vi "AccelerometerSample6.vi"(0 "Output type":i16=1, 1 "Period (ms)":i32=5) -> (2 "Ticks":u64, 3 "FIFO full":bool, 4 "Timeouted":bool)   [LabVIEW 2018]
uses:
  <vilib>/rvi/Emulation/niFpgaGetClockAttributes.vi
  <vilib>/rvi/Emulation/niFpgaSctlEmulationGetInTimedLoop.vi
  <vilib>/rvi/Emulation/niFpgaEmulationReportErrorSimple.vi
  <vilib>/rvi/eio/common/nirviEmuTemplateMethod_errors.vi
  <vilib>/rvi/occurrence/nirviWaitOnOccurrenceBase.vi
  <vilib>/rvi/Emulation/niFpgaCriticalErrorInLSC.vi
  <vilib>/rvi/Emulation/niFpgaProcessEmulError.vi
  <vilib>/eio/EIONode/EIONode.xnode
  <vilib>/eio/EIOMethodNode/EIOMethodNode.xnode
panel:
  # "Collects accelerometers data.\n\nValid data are written onto\n\"Output\" queue. If trigger isn't\nwithin \"Period\" milliseconds, timeout\n(\"Timeouted\") is signalized.\n\nStops collection when \"Stop\" GFV\nbecomes true. Writes current ticks\ninto \"Ticks register\" and on \"Ticks\"\noutput."
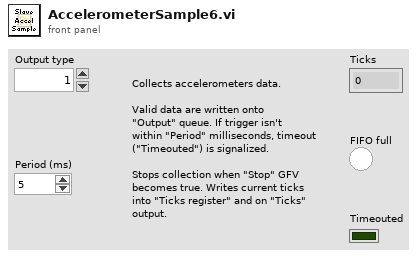
[diagram p1: front panel]
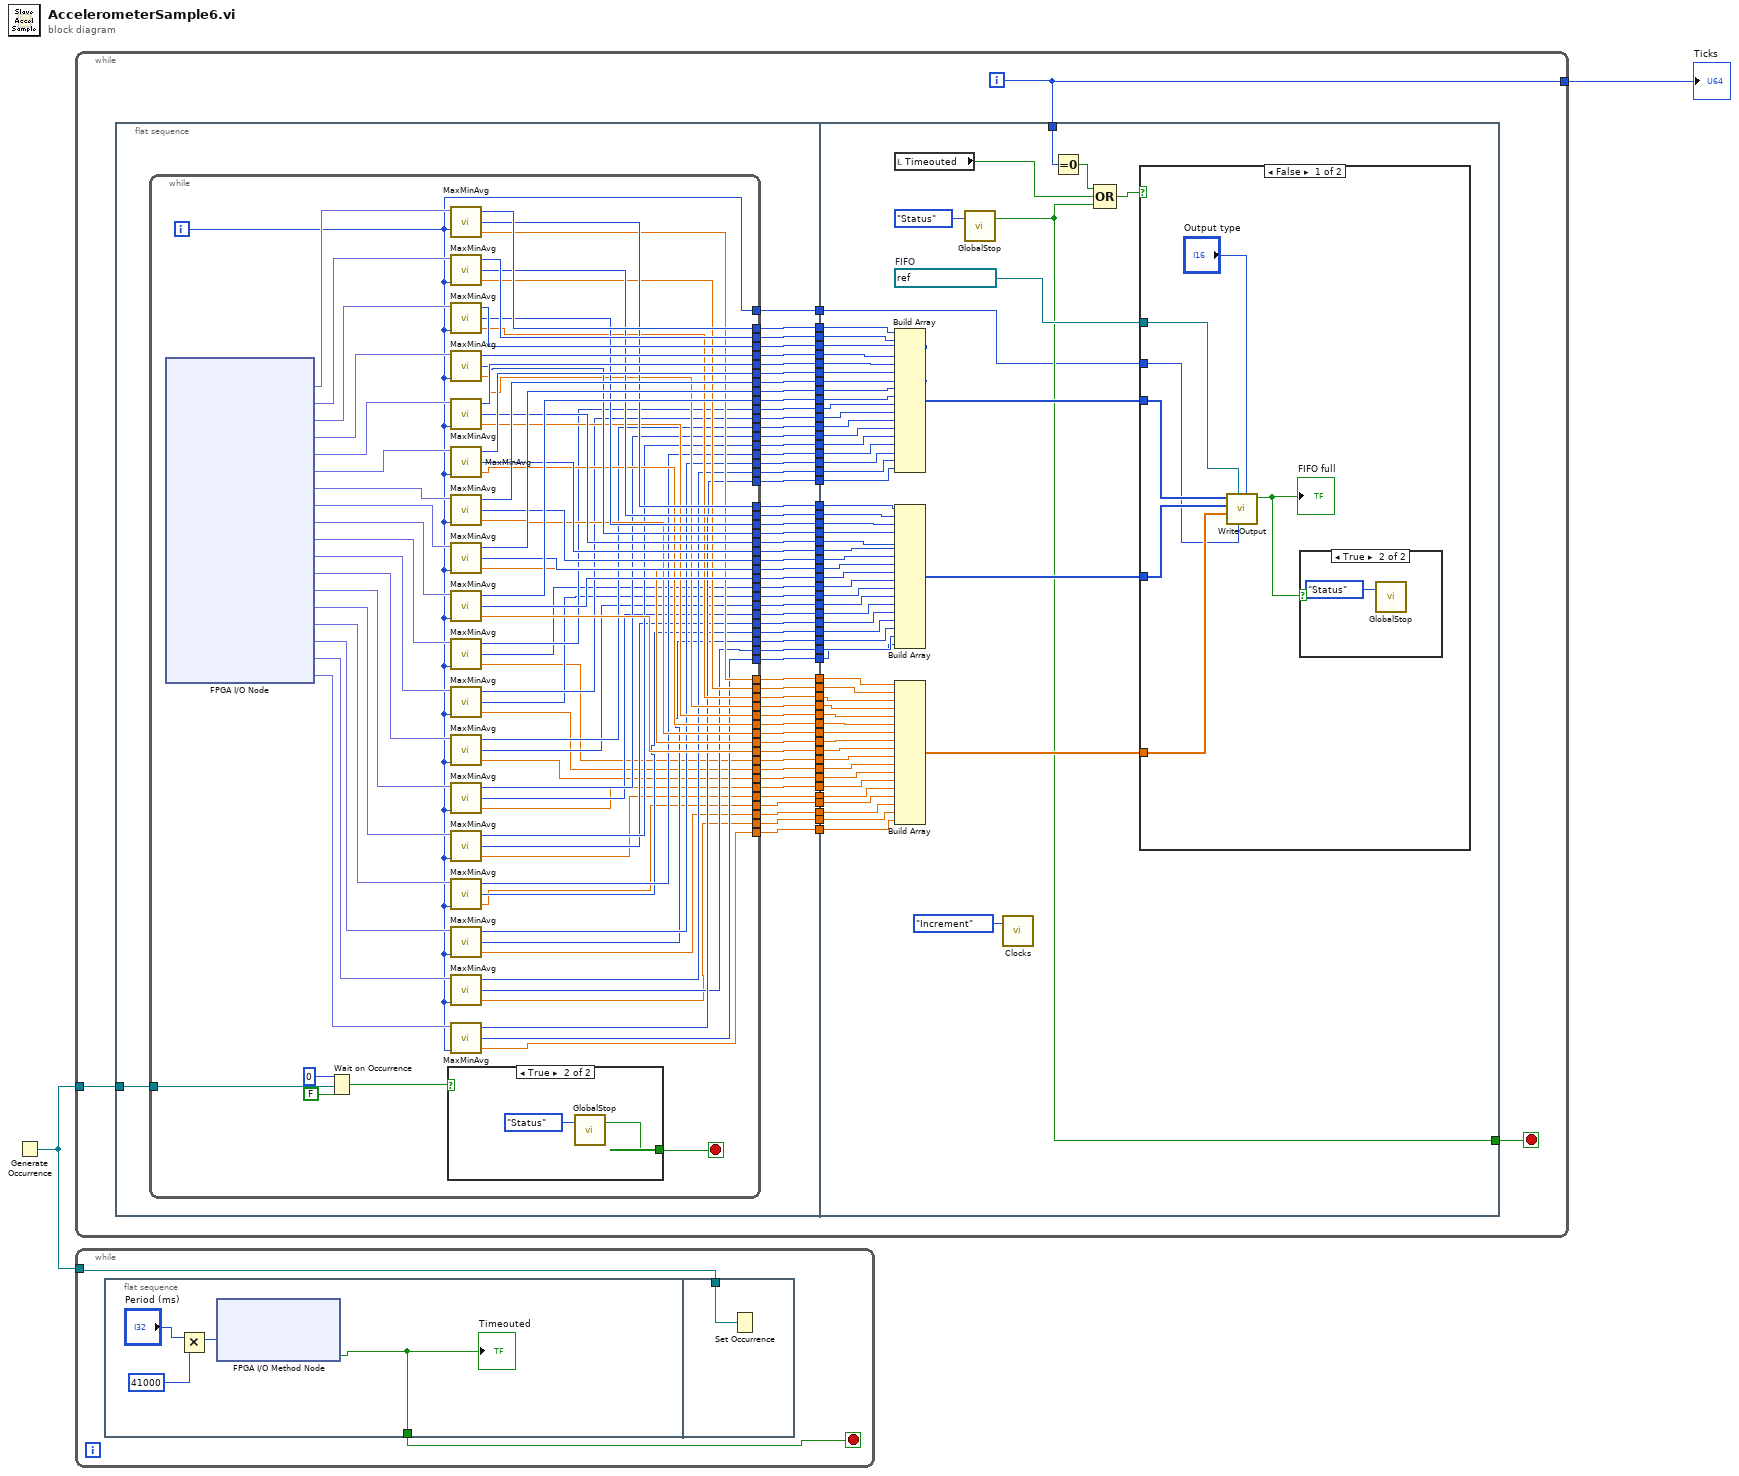
[diagram p0: block diagram]
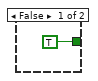
[diagram p2: hidden frame]
diagram:
  n1 = Generate Occurrence() -> (w2:refnum<k4>)
  n2 = while {
    tunnel: w2 -> [w34]
    tunnel: [w4] -> w1
    i -> [w4]
    stop <- w33 stop-if-true
    n3 = flat-sequence {
      tunnel: w34 -> [w116]
      tunnel: [w115] -> w60
      tunnel: [w114] -> w59
      tunnel: [w113] -> w58
      tunnel: [w112] -> w57
      tunnel: [w111] -> w56
      tunnel: [w110] -> w55
      tunnel: [w109] -> w54
      tunnel: [w108] -> w53
      tunnel: [w107] -> w52
      tunnel: [w106] -> w51
      tunnel: [w105] -> w50
      tunnel: [w104] -> w49
      tunnel: [w103] -> w48
      tunnel: [w102] -> w47
      tunnel: [w101] -> w46
      tunnel: [w100] -> w45
      tunnel: [w99] -> w44
      tunnel: [w98] -> w43
      tunnel: [w97] -> w42
      tunnel: [w96] -> w41
      tunnel: [w95] -> w40
      tunnel: [w94] -> w39
      tunnel: [w68] -> w38
      tunnel: [w93] -> w37
      tunnel: [w92] -> w36
      tunnel: [w91] -> w35
      tunnel: [w90] -> w32
      tunnel: [w89] -> w31
      tunnel: [w88] -> w30
      tunnel: [w87] -> w29
      tunnel: [w86] -> w28
      tunnel: [w85] -> w27
      tunnel: [w84] -> w26
      tunnel: [w83] -> w25
      tunnel: [w82] -> w24
      tunnel: [w81] -> w23
      tunnel: [w80] -> w22
      tunnel: [w79] -> w21
      tunnel: [w78] -> w20
      tunnel: [w77] -> w19
      tunnel: [w76] -> w18
      tunnel: [w75] -> w17
      tunnel: [w74] -> w16
      tunnel: [w73] -> w15
      tunnel: [w72] -> w14
      tunnel: [w71] -> w13
      tunnel: [w70] -> w12
      tunnel: [w69] -> w11
      tunnel: [w67] -> w10
      tunnel: [w66] -> w9
      tunnel: [w65] -> w8
      tunnel: [w64] -> w7
      tunnel: [w63] -> w6
      tunnel: [w62] -> w5
      tunnel: [w61] -> w3
      tunnel: w60 -> [w263]
      tunnel: w59 -> [w262]
      tunnel: w58 -> [w261]
      tunnel: w57 -> [w260]
      tunnel: w56 -> [w259]
      tunnel: w55 -> [w258]
      tunnel: w54 -> [w257]
      tunnel: w53 -> [w256]
      tunnel: w52 -> [w255]
      tunnel: w51 -> [w254]
      tunnel: w50 -> [w253]
      tunnel: w49 -> [w252]
      tunnel: w48 -> [w251]
      tunnel: w47 -> [w250]
      tunnel: w46 -> [w249]
      tunnel: w45 -> [w248]
      tunnel: w44 -> [w247]
      tunnel: w43 -> [w246]
      tunnel: w42 -> [w245]
      tunnel: w41 -> [w244]
      tunnel: w40 -> [w243]
      tunnel: w39 -> [w242]
      tunnel: w38 -> [w238]
      tunnel: w37 -> [w241]
      tunnel: w36 -> [w240]
      tunnel: w35 -> [w239]
      tunnel: [w201] -> w33
      tunnel: w32 -> [w233]
      tunnel: w31 -> [w232]
      tunnel: w30 -> [w231]
      tunnel: w29 -> [w230]
      tunnel: w28 -> [w229]
      tunnel: w27 -> [w228]
      tunnel: w26 -> [w227]
      tunnel: w25 -> [w226]
      tunnel: w24 -> [w225]
      tunnel: w23 -> [w224]
      tunnel: w22 -> [w223]
      tunnel: w21 -> [w222]
      tunnel: w20 -> [w221]
      tunnel: w19 -> [w220]
      tunnel: w18 -> [w219]
      tunnel: w17 -> [w218]
      tunnel: w16 -> [w217]
      tunnel: w15 -> [w216]
      tunnel: w14 -> [w215]
      tunnel: w13 -> [w214]
      tunnel: w12 -> [w213]
      tunnel: w11 -> [w212]
      tunnel: w10 -> [w211]
      tunnel: w9 -> [w210]
      tunnel: w8 -> [w209]
      tunnel: w7 -> [w208]
      tunnel: w6 -> [w207]
      tunnel: w5 -> [w206]
      tunnel: w4 -> [w200]
      tunnel: w3 -> [w198]
      frame #0 {
        n4 = while {
          tunnel: w116 -> [w194]
          tunnel: [w182] -> w115
          tunnel: [w181] -> w114
          tunnel: [w180] -> w113
          tunnel: [w179] -> w112
          tunnel: [w178] -> w111
          tunnel: [w177] -> w110
          tunnel: [w176] -> w109
          tunnel: [w175] -> w108
          tunnel: [w174] -> w107
          tunnel: [w173] -> w106
          tunnel: [w172] -> w105
          tunnel: [w171] -> w104
          tunnel: [w170] -> w103
          tunnel: [w169] -> w102
          tunnel: [w168] -> w101
          tunnel: [w167] -> w100
          tunnel: [w166] -> w99
          tunnel: [w165] -> w98
          tunnel: [w164] -> w97
          tunnel: [w163] -> w96
          tunnel: [w162] -> w95
          tunnel: [w161] -> w94
          tunnel: [w160] -> w68
          tunnel: [w159] -> w67
          tunnel: [w158] -> w93
          tunnel: [w157] -> w92
          tunnel: [w156] -> w91
          tunnel: [w146] -> w90
          tunnel: [w145] -> w89
          tunnel: [w144] -> w88
          tunnel: [w143] -> w87
          tunnel: [w142] -> w86
          tunnel: [w141] -> w85
          tunnel: [w140] -> w84
          tunnel: [w139] -> w83
          tunnel: [w138] -> w82
          tunnel: [w137] -> w81
          tunnel: [w136] -> w80
          tunnel: [w135] -> w79
          tunnel: [w134] -> w78
          tunnel: [w133] -> w77
          tunnel: [w132] -> w76
          tunnel: [w131] -> w75
          tunnel: [w130] -> w74
          tunnel: [w129] -> w73
          tunnel: [w128] -> w72
          tunnel: [w127] -> w71
          tunnel: [w126] -> w70
          tunnel: [w125] -> w69
          tunnel: [w124] -> w66
          tunnel: [w123] -> w65
          tunnel: [w122] -> w64
          tunnel: [w121] -> w63
          tunnel: [w120] -> w62
          tunnel: [w117] -> w61
          i -> [w117]
          stop <- w119 stop-if-true
          n5 = xnode "FPGA I/O Node"() -> ("Accelerometer1/AI0"=w191:fxp<+/-,24,7>, "Accelerometer1/AI1"=w190:fxp<+/-,24,7>, "Accelerometer1/AI2"=w189:fxp<+/-,24,7>, "Accelerometer2/AI0"=w188:fxp<+/-,24,7>, "Accelerometer2/AI1"=w187:fxp<+/-,24,7>, "Accelerometer2/AI2"=w186:fxp<+/-,24,7>, "Accelerometer3/AI0"=w185:fxp<+/-,24,7>, "Accelerometer3/AI1"=w184:fxp<+/-,24,7>, "Accelerometer3/AI2"=w183:fxp<+/-,24,7>, "Accelerometer4/AI0"=w155:fxp<+/-,24,7>, "Accelerometer4/AI1"=w154:fxp<+/-,24,7>, "Accelerometer4/AI2"=w153:fxp<+/-,24,7>, "Accelerometer5/AI0"=w152:fxp<+/-,24,7>, "Accelerometer5/AI1"=w151:fxp<+/-,24,7>, "Accelerometer5/AI2"=w150:fxp<+/-,24,7>, "Accelerometer6/AI0"=w149:fxp<+/-,24,7>, "Accelerometer6/AI1"=w148:fxp<+/-,24,7>, "Accelerometer6/AI2"=w147:fxp<+/-,24,7>)  [unwired: 18 in, 18 out]
          n6 = Wait on Occurrence(1:FALSE ("ignore previous (T)"), 2:w194, 3:0 ("ms timeout (-1)")) -> (0:w118:bool)
          n7 = case shown="True" w118 {
            tunnel: [TRUE w196] -> w119
            frame False {
            }
            frame True {
              n8 = call "GlobalStop.vi"("Enum"=enum16{"Clear", "Set", "Status"}."Status") -> ("Boolean"=w196:bool)  [unwired: 1 in, 1 out]
            }
          }
          n9 = call "MaxMinAvg.vi"("Index"=w117, "Measurement"=w191) -> ("Average Value"=w164:sgl, "Minimum Value"=w173:i32, "Maximum Value"=w182:i32)  [unwired: 2 in]
          n10 = call "MaxMinAvg.vi"("Index"=w117, "Measurement"=w190) -> ("Average Value"=w163:sgl, "Minimum Value"=w172:i32, "Maximum Value"=w181:i32)  [unwired: 2 in]
          n11 = call "MaxMinAvg.vi"("Index"=w117, "Measurement"=w189) -> ("Average Value"=w162:sgl, "Minimum Value"=w171:i32, "Maximum Value"=w180:i32)  [unwired: 2 in]
          n12 = call "MaxMinAvg.vi"("Index"=w117, "Measurement"=w188) -> ("Average Value"=w161:sgl, "Minimum Value"=w170:i32, "Maximum Value"=w179:i32)  [unwired: 2 in]
          n13 = call "MaxMinAvg.vi"("Index"=w117, "Measurement"=w187) -> ("Average Value"=w160:sgl, "Minimum Value"=w169:i32, "Maximum Value"=w178:i32)  [unwired: 2 in]
          n14 = call "MaxMinAvg.vi"("Index"=w117, "Measurement"=w186) -> ("Average Value"=w159:sgl, "Minimum Value"=w168:i32, "Maximum Value"=w177:i32)  [unwired: 2 in]
          n15 = call "MaxMinAvg.vi"("Index"=w117, "Measurement"=w185) -> ("Average Value"=w158:sgl, "Minimum Value"=w167:i32, "Maximum Value"=w176:i32)  [unwired: 2 in]
          n16 = call "MaxMinAvg.vi"("Index"=w117, "Measurement"=w184) -> ("Average Value"=w157:sgl, "Minimum Value"=w166:i32, "Maximum Value"=w175:i32)  [unwired: 2 in]
          n17 = call "MaxMinAvg.vi"("Index"=w117, "Measurement"=w183) -> ("Average Value"=w156:sgl, "Minimum Value"=w165:i32, "Maximum Value"=w174:i32)  [unwired: 2 in]
          n18 = call "MaxMinAvg.vi"("Index"=w117, "Measurement"=w155) -> ("Average Value"=w128:sgl, "Minimum Value"=w137:i32, "Maximum Value"=w146:i32)  [unwired: 2 in]
          n19 = call "MaxMinAvg.vi"("Index"=w117, "Measurement"=w154) -> ("Average Value"=w127:sgl, "Minimum Value"=w136:i32, "Maximum Value"=w145:i32)  [unwired: 2 in]
          n20 = call "MaxMinAvg.vi"("Index"=w117, "Measurement"=w153) -> ("Average Value"=w126:sgl, "Minimum Value"=w135:i32, "Maximum Value"=w144:i32)  [unwired: 2 in]
          n21 = call "MaxMinAvg.vi"("Index"=w117, "Measurement"=w152) -> ("Average Value"=w125:sgl, "Minimum Value"=w134:i32, "Maximum Value"=w143:i32)  [unwired: 2 in]
          n22 = call "MaxMinAvg.vi"("Index"=w117, "Measurement"=w151) -> ("Average Value"=w124:sgl, "Minimum Value"=w133:i32, "Maximum Value"=w142:i32)  [unwired: 2 in]
          n23 = call "MaxMinAvg.vi"("Index"=w117, "Measurement"=w150) -> ("Average Value"=w123:sgl, "Minimum Value"=w132:i32, "Maximum Value"=w141:i32)  [unwired: 2 in]
          n24 = call "MaxMinAvg.vi"("Index"=w117, "Measurement"=w149) -> ("Average Value"=w122:sgl, "Minimum Value"=w131:i32, "Maximum Value"=w140:i32)  [unwired: 2 in]
          n25 = call "MaxMinAvg.vi"("Index"=w117, "Measurement"=w148) -> ("Average Value"=w121:sgl, "Minimum Value"=w130:i32, "Maximum Value"=w139:i32)  [unwired: 2 in]
          n26 = call "MaxMinAvg.vi"("Index"=w117, "Measurement"=w147) -> ("Average Value"=w120:sgl, "Minimum Value"=w129:i32, "Maximum Value"=w138:i32)  [unwired: 2 in]
        }
      }
      frame #1 {
        w237 = refnum<k21> "ResponseFIFO"  # FIFO
        n27 = local read "Timeouted"() -> (w203:bool)
        n28 = Build Array(w263, w262, w261, w260, w259, w258, w257, w256, w255, w233, w232, w231, w230, w229, w228, w227, w226, w225) -> (w236:i32[])
        n29 = Build Array(w254, w253, w252, w251, w250, w249, w248, w247, w246, w224, w223, w222, w221, w220, w219, w218, w217, w216) -> (w235:i32[])
        n30 = Build Array(w245, w244, w243, w242, w238, w211, w241, w240, w239, w215, w214, w213, w212, w210, w209, w208, w207, w206) -> (w234:sgl[])
        n31 = call "GlobalStop.vi"("Enum"=enum16{"Clear", "Set", "Status"}."Status") -> ("Boolean"=w201:bool)  [unwired: 1 in, 1 out]
        n32 = call "Clocks.vi"("Enum"=enum16{"Reset", "Increment", "Get"}."Increment") -> ()  [unwired: 1 in, 2 out]
        n33 = Equal To 0?(x=w200) -> (x = 0?=w204:bool)
        n34 = Compound Arithmetic op=OR(w204, w203, w201) -> (w205:bool)
        n35 = case shown="False" w205 {
          tunnel: w237 -> [w270 _]
          tunnel: w236 -> [w269 _]
          tunnel: w235 -> [w268 _]
          tunnel: w234 -> [w267 _]
          tunnel: w198 -> [w265 _]
          frame False {
            n36 = call "WriteOutput.vi"("Output type"="Output type", "Number of Samples"=w265, "Output FIFO"=w270, "Average"=w267, "Max"=w268, "Min"=w269) -> ("FIFO full"=w264:bool)  [unwired: 5 in]
            "FIFO full" <- w264
            n37 = case shown="True" w264 {
              frame False {
              }
              frame True {
                n38 = call "GlobalStop.vi"("Enum"=enum16{"Clear", "Set", "Status"}."Status") -> ()  [unwired: 1 in, 2 out]
              }
            }
          }
          frame True {
          }
        }
      }
    }
  }
  "Ticks" <- w1
  n39 = while {
    tunnel: w2 -> [w273]
    stop <- w272 stop-if-true
    n40 = flat-sequence {
      tunnel: [w274] -> w272
      tunnel: w273 -> [w278]
      frame #0 {
        n41 = Multiply(x="Period (ms)", y=41000) -> (x*y=w277:i32)
        n42 = xnode "FPGA I/O Method Node"("Timeout"=w277) -> ("Timed Out"=w274:bool)  [unwired: 1 in, 1 out]
        "Timeouted" <- w274
      }
      frame #1 {
        n43 = Set Occurrence(w278) -> ()
      }
    }
  }
